vi "TCPListenMulligan.vi"(8 "error in (no error)":errorcluster) -> (0 "error out":errorcluster, 3 "listener ID":refnum<k5>)   [LabVIEW 2013]
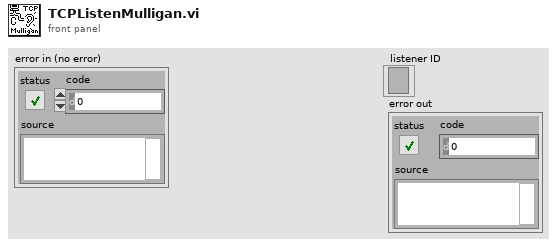
[diagram p1: front panel]
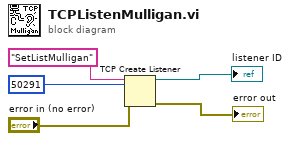
[diagram p0: block diagram]
diagram:
  n1 = TCP Create Listener(8:"error in (no error)", 10:u16 50291 ("port"), 11:"SetListMulligan" ("service name")) -> (0:→"error out":errorcluster, 3:→"listener ID":refnum<k5>)  [unwired: 2 in, 1 out]
